vi "ErrorHandling.vi"(8 "error in (no error)":errorcluster, 10 "stop":bool, 11 "Emergency Button":bool) -> (3 "Boolean":bool)   [LabVIEW 2013]
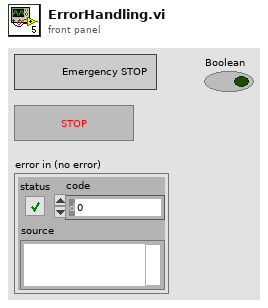
[diagram p1: front panel]
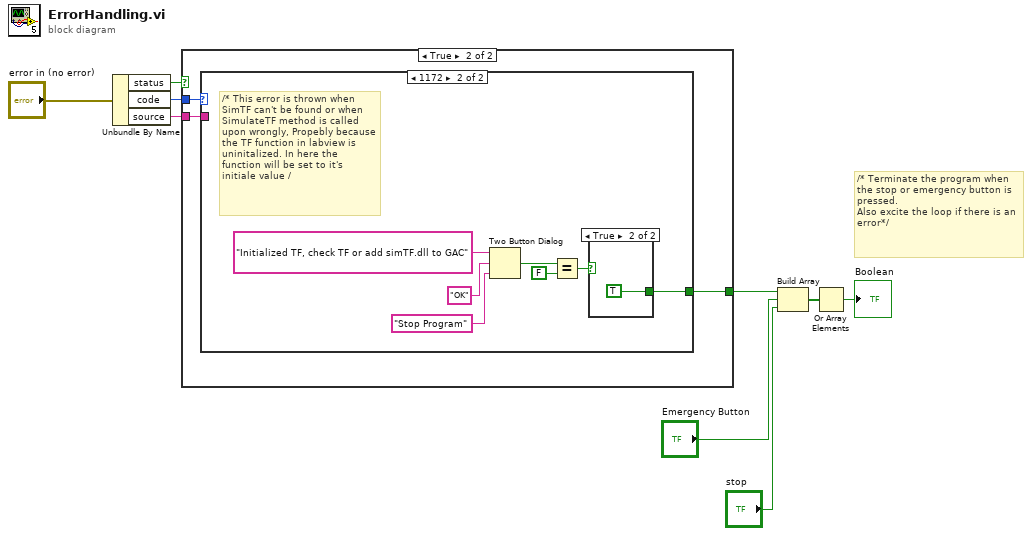
[diagram p0: block diagram]
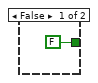
[diagram p2: hidden frame]
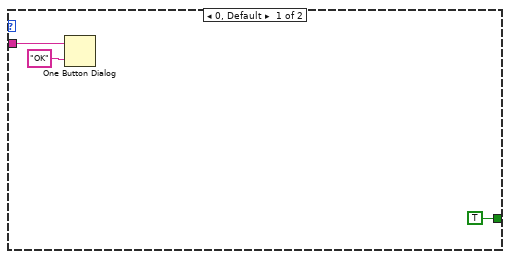
[diagram p3: hidden frame]
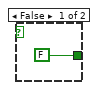
[diagram p4: hidden frame]
diagram:
  # "/* Terminate the program when the stop or emergency button is pressed.  \nAlso excite the loop if there is an error*/"
  n1 = Unbundle By Name("error in (no error)") -> ("status"=w9:bool, "code"=w4:i32, "source"=w5:string)
  n2 = case shown="True" w9 {
    tunnel: w4 -> [_ w13]
    tunnel: w5 -> [_ w12]
    tunnel: [FALSE w11] -> w6
    frame False {
    }
    frame True {
      n3 = case shown="1172" w13 {
        tunnel: w12 -> [w15 _]
        tunnel: [TRUE w17] -> w11
        frame 0, Default {
          n4 = One Button Dialog(message=w15, button name ("OK")="OK") -> ()  [unwired: 1 out]
        }
        frame 1172 {
          # "/* This error is thrown when SimTF can't be found or when SimulateTF method is called upon wrongly, Propebly because the TF function in labview is uninitalized. In here the function will be set to it's initiale value /"
          n5 = Two Button Dialog(message="Initialized TF, check TF or add simTF.dll to GAC", 1:"Stop Program" ("F button name (\"Cancel\")"), 2:"OK" ("button name (\"OK\")")) -> (T button?=w20:bool)
          n6 = Equal?(x=w20, y=FALSE) -> (x = y?=w18:bool)
          n7 = case shown="True" w18 {
            tunnel: [FALSE TRUE] -> w17
            frame False {
            }
            frame True {
            }
          }
        }
      }
    }
  }
  n8 = Build Array(w6, "Emergency Button", "stop") -> (w8:bool[])
  n9 = Or Array Elements(Boolean array=w8) -> (logical OR=→"Boolean":bool)
